vi "Project Spec Type.vi"(0 "NI Build Specification in":refnum<class "SourceDist_LV.lvclass">, 11 "error in (no error)":errorcluster) -> (4 "NI Build Specification out":refnum<class "SourceDist_LV.lvclass">, 6 "Project Specfication Type":string, 15 "error out":errorcluster)   [LabVIEW 2017, in "CL_G3_VIComponentBuilder.lvlib" / "SourceDist_LV.lvclass"]
doc: "Returns the type of the build specification for a source distribution."
uses:
  SourceDist_LV.lvclass
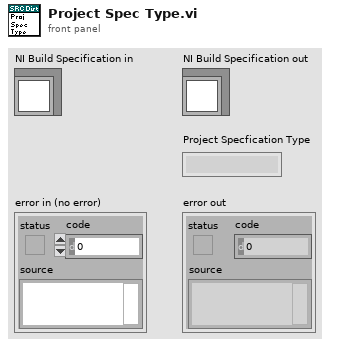
[diagram p1: front panel]
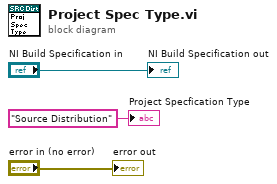
[diagram p0: block diagram]
diagram:
  "error out" <- "error in (no error)"
  "NI Build Specification out" <- "NI Build Specification in"
  "Project Specfication Type" <- "Source Distribution" ("Project Specfication Type")
